vi "Release-user-events.vi"(8 "error in (no error)":errorcluster, 11 "ModComm in":T1) -> (0 "error out":errorcluster, 3 "ModComm out":T1)   [LabVIEW 2013, in "SLMServer.lvlib" / "SLMServer.lvclass"]
uses:
  SLMServer.lvclass
  Object-reference.ctl
  SLMServer.lvclass/SLMServer.ctl
  Read Activity log.vi
  Read Error log.vi
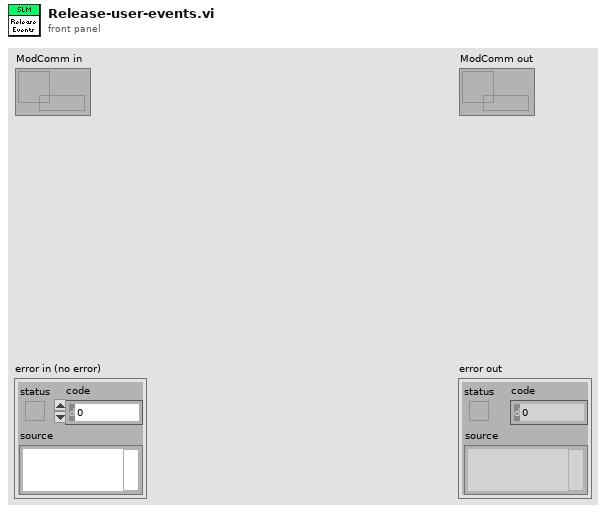
[diagram p1: front panel]
types:
  T1 = typedef "SLMServer.lvlib/SLMServer.lvclass/Object-reference.ctl" = refnum<data-value>
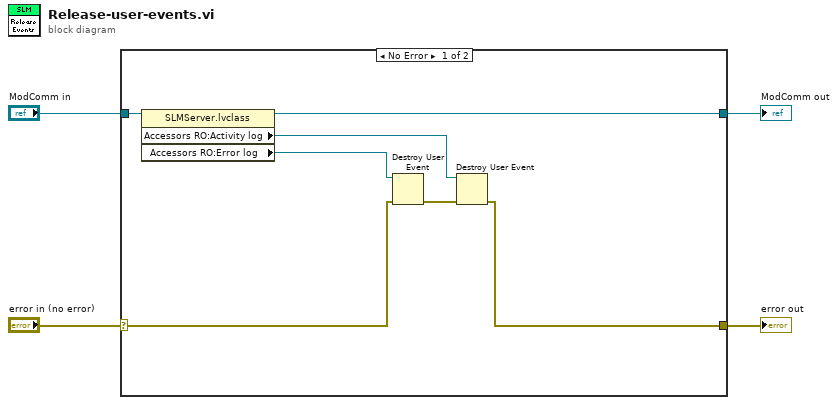
[diagram p0: block diagram]
diagram:
  n1 = case shown="No Error" "error in (no error)" {
    selector: "error in (no error)" -> [w5 w13]
    tunnel: [w7 w13] -> w3
    tunnel: [w10 w12] -> w1
    tunnel: "ModComm in" -> [w11 w12]
    frame No Error {
      n2 = property class="SLMServer.lvclass"(reference=w11) -> (reference out=w10:T1, "Accessors RO:Activity log"=w9:refnum<user-event>, "Accessors RO:Error log"=w8:refnum<user-event>)  [unwired: 1 in, 1 out]
      n3 = Destroy User Event(user event=w8, error in=w5) -> (error out=w6:errorcluster)
      n4 = Destroy User Event(user event=w9, error in=w6) -> (error out=w7:errorcluster)
    }
    frame Error {
    }
  }
  "error out" <- w3
  "ModComm out" <- w1
